vi "VI Template Launcher.vi"   [LabVIEW 2011]
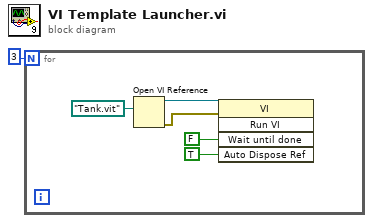
[diagram p0: block diagram]
diagram:
  n1 = for {
    N: 3 -> [_]
    n2 = Open VI Reference(vi path=path "Tank.vit") -> (vi reference=w3:refnum<vi>, error out=w2:errorcluster)  [unwired: 5 in]
    n3 = invoke class="VI" method="Run VI"(reference=w3, error in=w2, "Wait until done"=FALSE ("Wait Until Done"), "Auto Dispose Ref"=TRUE ("Auto Dispose Reference")) -> ()  [unwired: 1 in, 5 out]
  }
